vi "ScanAction.vi"(8 "error in (no error)":errorcluster caption="entrée d'erreur (pas d'erreur)", 9 "IndicePoint":i32, 10 "Dir":bool, 11 "AppliedMoitionDrive In":refnum<class "AppliedMotionDrive.lvclass"> caption="DNL_LabVIEW Object in") -> (0 "error out":errorcluster caption="sortie d'erreur", 2 "ScanParsOut":dbl[](array[numeric]), 3 "AppliedMotionDrive Out":refnum<class "AppliedMotionDrive.lvclass"> caption="DNL_LabVIEW Object out")   [LabVIEW 2019, in "AppliedMotionDrive.lvclass"]
uses:
  AppliedMotionDrive.lvclass
  C:/Programmes Labview/LabscanV1A/DevicesClass/BaseDevice/BaseDevice.lvclass
  AppliedMotionDrive.lvclass/AppliedMotionDrive.ctl
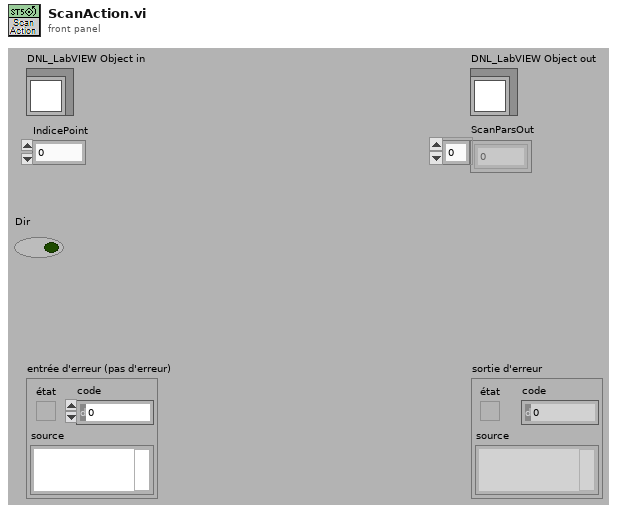
[diagram p1: front panel]
types:
  T1 = typedef "AppliedMotionDrive.lvclass/AppliedMotionDrive_Func.ctl" = enum16{"Position (Units)", "FilterWheel (Id)"}
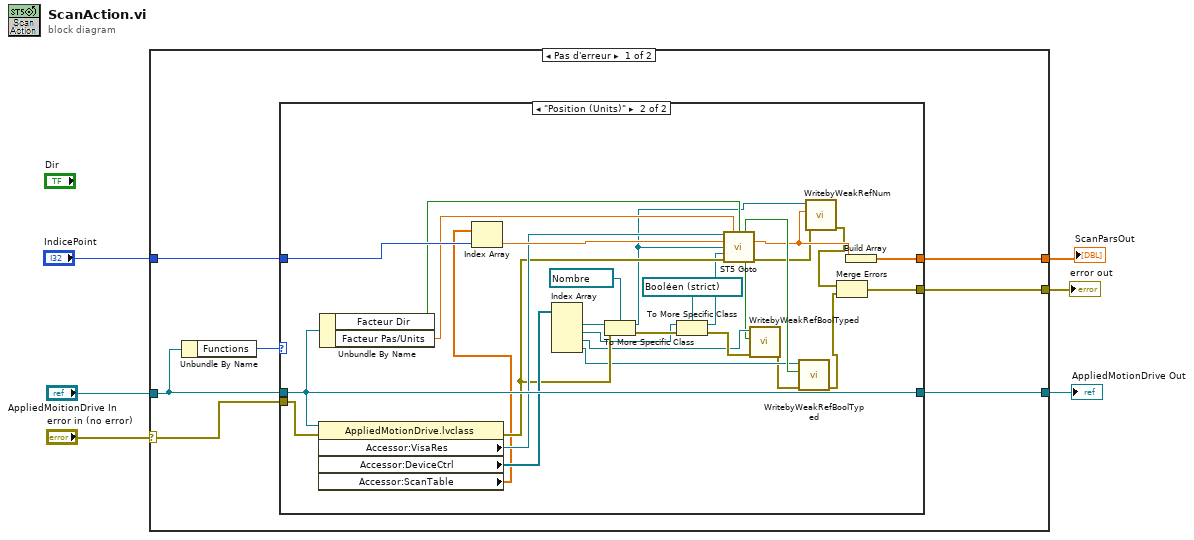
[diagram p0: block diagram]
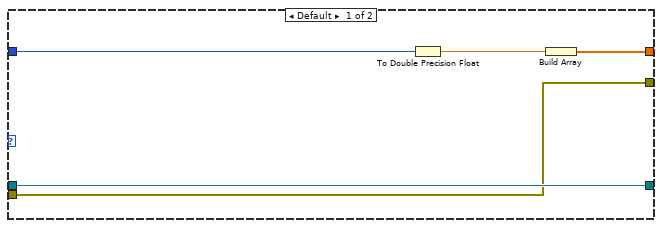
[diagram p2: hidden frame]
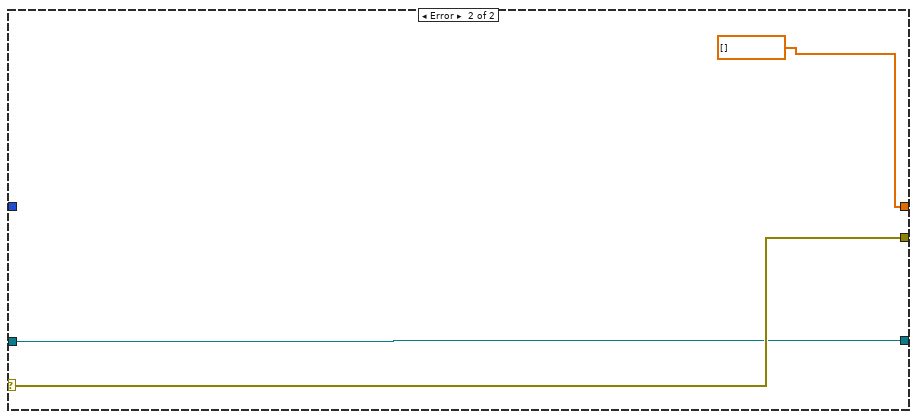
[diagram p3: hidden frame]
diagram:
  n1 = case shown="Pas d'erreur" "error in (no error)" {
    selector: "error in (no error)" -> [w10 w50]
    tunnel: "AppliedMoitionDrive In" -> [w11 w49]
    tunnel: [w9 dbl[] []] -> w1
    tunnel: [w8 w50] -> w4
    tunnel: [w7 w49] -> w3
    tunnel: "IndicePoint" -> [w12 _]
    frame No Error {
      n2 = Unbundle By Name(w11) -> ("Functions"=w13:T1)
      n3 = case shown="\"Position (Units)\"" w13 {
        tunnel: [w14 w19] -> w9
        tunnel: w12 -> [w18 w47]
        tunnel: [w16 w45] -> w7
        tunnel: w11 -> [w16 w45]
        tunnel: w10 -> [w15 w43]
        tunnel: [w15 w38] -> w8
        frame Default {
          n4 = To Double Precision Float(number=w18) -> (double precision float=w17:dbl)
          n5 = Build Array(w17) -> (w14:dbl[])
        }
        frame "Position (Units)" {
          n6 = property class="AppliedMotionDrive.lvclass"(reference=w45, error in=w43) -> (error out=w39:errorcluster, "Accessor:VisaRes"=w44:refnum<visa-resource-name>, "Accessor:DeviceCtrl"=w40:refnum<vi>[], "Accessor:ScanTable"=w24:dbl[])  [unwired: 1 out]
          n7 = Unbundle By Name(w45) -> ("Facteur Dir"=w41:bool, "Facteur Pas/Units"=w42:dbl)
          n8 = Index Array(array=w24, index=w47) -> (element=w46:dbl)
          n9 = Index Array(array=w40) -> (element #1=w29:refnum<vi>, element #2=w25:refnum<vi>, element #3=w32:refnum<vi>, element #4=w36:refnum<vi>)  [unwired: 4 in]
          n10 = To More Specific Class(target class=refnum<vi> refnum ("Stop Ref"), reference=w29, error in=w39) -> (specific class reference=w22:refnum<vi>, error out=w35:errorcluster)
          n11 = To More Specific Class(target class=refnum<vi> refnum ("Stop Ref"), reference=w25, error in=w35) -> (specific class reference=w27:refnum<vi>, error out=w34:errorcluster)
          n12 = call <userlib>:"ST5 Goto.vi"("Port COM"=w44, "Facteur Pas"=w42, "Facteur Dir"=w41, "Position"=w46, "PositionRef"=w22, "Ext Stop Ref"=w27, "error in (no error)"=w39) -> ("CCW Limit"=w37:bool, "Position Out"=w23:dbl, "CW Limit"=w30:bool, "error out"=w21:errorcluster)  [unwired: 2 in, 3 out]
          n13 = call <userlib>:"WritebyWeakRefBoolTyped.vi"("error in"=w34, "Valeur"=w30, "Control Ref"=w32) -> ("error out"=w31:errorcluster)  [unwired: 8 in]
          n14 = call <userlib>:"WritebyWeakRefBoolTyped.vi"("error in"=w31, "Valeur"=w37, "Control Ref"=w36) -> ("error out"=w33:errorcluster)  [unwired: 8 in]
          n15 = call <userlib>:"WritebyWeakRefNum.vi"("error in"=w21, "Valeur"=w23, "Control Ref"=w22) -> ("error out"=w20:errorcluster)  [unwired: 8 in]
          n16 = Merge Errors(w20, w33) -> (w38:errorcluster)
          n17 = Build Array(w23) -> (w19:dbl[])
        }
      }
    }
    frame Error {
    }
  }
  "error out" <- w4
  "AppliedMotionDrive Out" <- w3
  "ScanParsOut" <- w1
